vi "clearFIFO.vi"(8 "error in (no error)":errorcluster, 11 "Mockbus in":refnum<class "Mockbus.lvclass">) -> (0 "error out":errorcluster, 3 "Mockbus out":refnum<class "Mockbus.lvclass">)   [LabVIEW 2015, in "Mockbus.lvclass"]
uses:
  Mockbus.lvclass
  Typedefs/Frame.ctl
  Mockbus.lvclass/Mockbus.ctl
  Typedefs/RTTypeDefs.lvlib
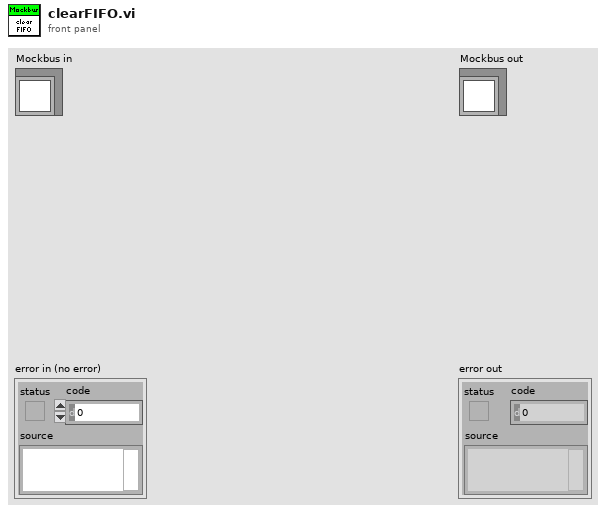
[diagram p1: front panel]
types:
  T1 = typedef "RTTypeDefs.lvlib/Frame.ctl" = cluster{"Data":u8[], "WaitForTrigger":bool, "WaitForRx":u16, "TriggerIRQ":i16}
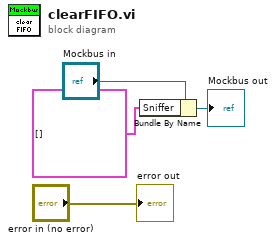
[diagram p0: block diagram]
diagram:
  n1 = Bundle By Name(cluster="Mockbus in", "Sniffer"=T1[] []) -> (→"Mockbus out":refnum<class "Mockbus.lvclass">)
  "error out" <- "error in (no error)"
